vi "22_waveform_chart_experiments.vi"() -> ()   [LabVIEW 2021]
panel:
  out "Waveform Chart":dynamicdata(graph)
  in  "stop":bool
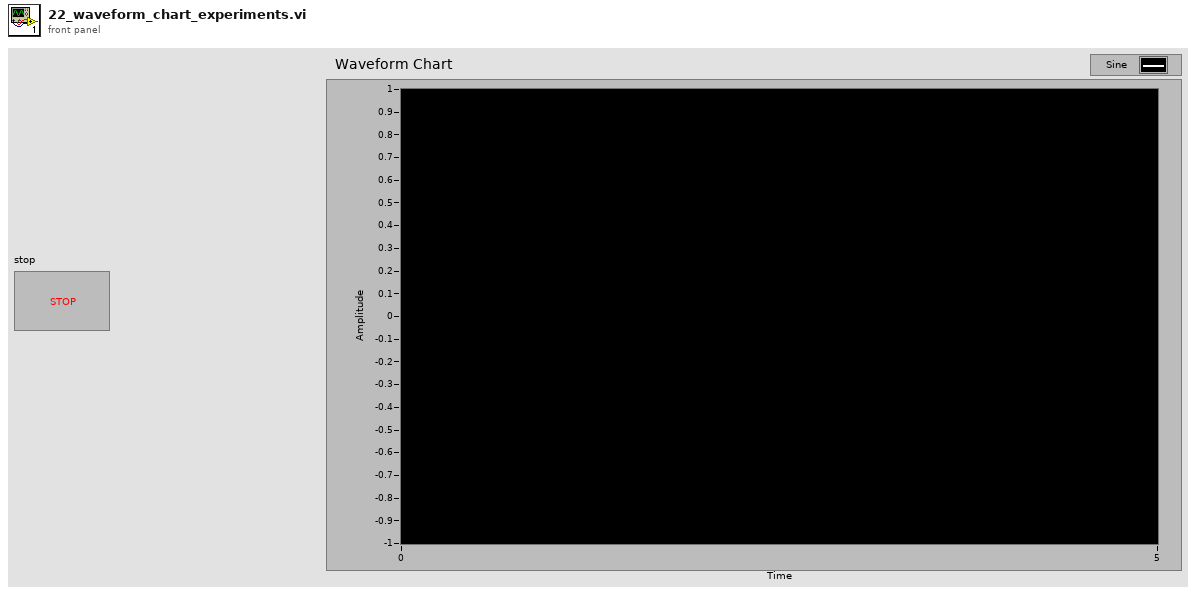
[diagram p1: front panel]
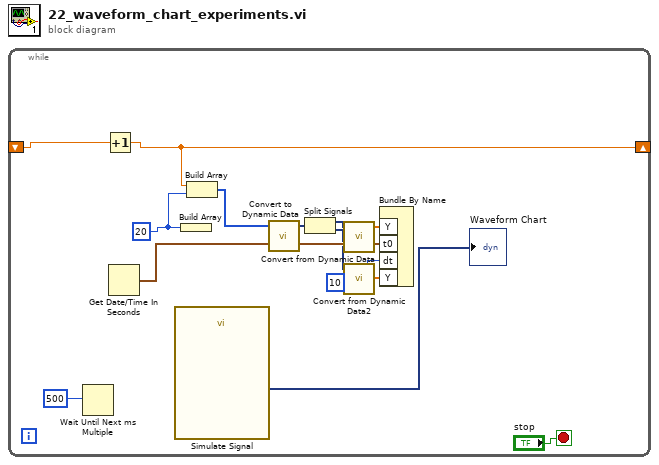
[diagram p0: block diagram]
diagram:
  n1 = while {
    shift-right: [w11] -> _
    shift-left: _ -> [w13]
    stop <- "stop" stop-if-true
    w8 = 20
    n2 = Wait Until Next ms Multiple(millisecond multiple=500) -> ()  [unwired: 1 out]
    n3 = Increment(x=w13) -> (x+1=w11:dbl)
    n4 = Get Date/Time In Seconds() -> (seconds since 1Jan1904=w10:timestamp)
    n5 = call "Simulate Signal"() -> ("Sine"=→"Waveform Chart":dynamicdata)  [unwired: 14 in, 1 out]
    n6 = Build Array(w8) -> ()  [unwired: 1 out]
    n7 = Build Array(w11, w8) -> (w7:i32[])
    n8 = call "Convert to Dynamic Data"("Array"=w7) -> ("Dynamic Data Type"=w6:dynamicdata)  [unwired: 3 in]
    n9 = Split Signals(w6) -> (w5:dynamicdata, w3:dynamicdata)  [unwired: 2 in]
    n10 = call "Convert from Dynamic Data"("Dynamic Data Type"=w5) -> ("Array"=w4:dbl[])  [unwired: 3 in]
    n11 = call "Convert from Dynamic Data2"("Dynamic Data Type"=w3) -> ("Array"=w2:dbl[])  [unwired: 3 in]
    n12 = Bundle By Name("Y"=w4, "t0"=w10, "dt"=10, "Y"=w2) -> ()  [unwired: 1 in, 1 out]
  }
